vi "executeDuelistSkill.vi"(8 "error in (no error)":errorcluster, 9 "Duelist Robot in":refnum<class "Robot.lvclass">, 10 "Game":refnum<class "Game.lvclass">, 11 "DuelistSkill in":refnum<class "DuelistSkill.lvclass">) -> (0 "error out":errorcluster, 1 "Duelist Robot out":refnum<class "Robot.lvclass">, 3 "DuelistSkill out":refnum<class "DuelistSkill.lvclass">)   [LabVIEW 2023, in "DuelistSkill.lvclass"]
uses:
  DuelistSkill.lvclass
  Utilities_class/Utilities.lvclass
  Game_class/Game.lvclass
  Enemy_class/Enemy.lvclass
  Robot_class/Robot.lvclass
  Field_class/Field.lvclass
  Ball_class/Ball.lvclass
  C:/Users/pedro/Desktop/SSL_AI/Object_class/Object.lvclass
  C:/Users/pedro/Desktop/SSL_AI/Ball_class/Ball.lvclass
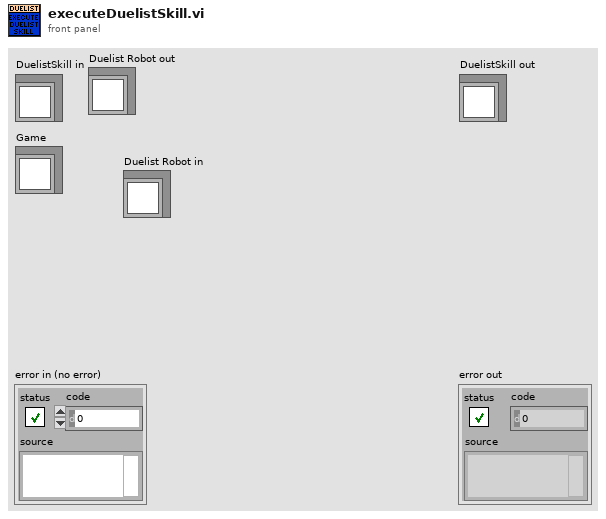
[diagram p1: front panel]
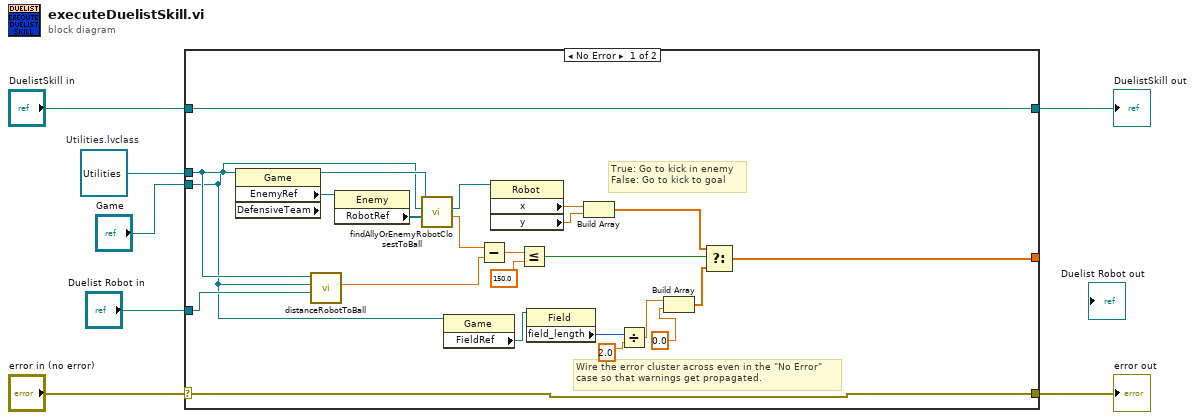
[diagram p0: block diagram]
diagram:
  w3 = refnum<class "Utilities.lvclass"> refnum  # Utilities.lvclass
  n1 = case shown="No Error" "error in (no error)" {
    selector: "error in (no error)" -> [w29 w32]
    tunnel: [w29 w32] -> w6
    tunnel: [w30 w31] -> w4
    tunnel: "DuelistSkill in" -> [w30 w31]
    tunnel: w3 -> [w26 _]
    tunnel: "Game" -> [w15 _]
    tunnel: "Duelist Robot in" -> [w25 _]
    tunnel: [w8 _] -> _
    frame No Error {
      # "True: Go to kick in enemy\nFalse: Go to kick to goal"
      # "Wire the error cluster across even in the \"No Error\"\ncase so that warnings get propagated."
      n2 = property class="Game" props=["EnemyRef", "DefensiveTeam"](reference=w15) -> ("EnemyRef"=w28:refnum<class "Enemy.lvclass">)  [unwired: 1 in, 3 out]
      n3 = call "distanceRobotToBall.vi"("Robot"=w25, "Ball"=w15, "Utilities in"=w26) -> ("Distance Robot To Ball"=w23:dbl)  [unwired: 6 in, 2 out]
      n4 = property class="Enemy"(reference=w28) -> ("RobotRef"=w27:refnum<class "Robot.lvclass">[])  [unwired: 1 in, 2 out]
      n5 = call "findAllyOrEnemyRobotClosestToBall.vi"("Ally/Enemy Robots"=w27, "Ball"=w15, "Utilities in"=w26) -> ("Robot distance to ball"=w24:dbl, "Robot"=w19:refnum<class "Robot.lvclass">)  [unwired: 5 in, 2 out]
      n6 = property class="Game"(reference=w15) -> ("FieldRef"=w14:refnum<class "Field.lvclass">)  [unwired: 1 in, 2 out]
      n7 = Subtract(x=w24, y=w23) -> (x-y=w22:dbl)
      n8 = property class="Robot"(reference=w19) -> ("x"=w18:dbl, "y"=w17:dbl)  [unwired: 1 in, 2 out]
      n9 = Less Or Equal?(x=w22, y=150.0) -> (x <= y?=w20:bool)
      n10 = property class="Field"(reference=w14) -> ("field_length"=w13:i32)  [unwired: 1 in, 2 out]
      n11 = Build Array(w18, w17) -> (w16:dbl[])
      n12 = Divide(x=w13, y=2.0 ("field_length")) -> (x/y=w11:dbl)
      n13 = Build Array(w11, 0.0 ("field_length")) -> (w9:dbl[])
      n14 = Select(t=w16, s=w20, f=w9) -> (s? t:f=w8:dbl[])
    }
    frame Error {
    }
  }
  "error out" <- w6
  "DuelistSkill out" <- w4
